vi "GET Save Directory.vi"() -> (0 "Save Directory":path)   [LabVIEW 2013]
uses:
  Action.ctl
  Persistent Data FGV Selector.ctl
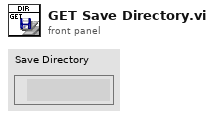
[diagram p1: front panel]
types:
  T1 = typedef "Persistent Data FGV Selector.ctl" = enum16{"Save Directory", "File Name"}
  T2 = typedef "Action.ctl" = enum16{"GET", "PUT", "DELETE"}
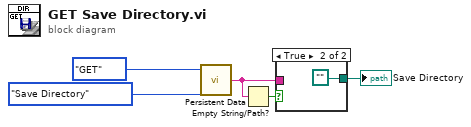
[diagram p0: block diagram]
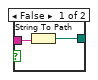
[diagram p2: hidden frame]
diagram:
  n1 = call "Persistent Data.vi"("Persistent Data FGV Selector"=Persistent_Data_FGV_Selector."Save Directory", "Action"=Action."GET") -> ("Output"=w1:string)  [unwired: 1 in]
  n2 = Empty String/Path?(string/path=w1) -> (empty?=w2:bool)
  n3 = case shown="True" w2 {
    tunnel: w1 -> [w7 _]
    tunnel: [w6 path ""] -> w3
    frame False {
      n4 = String To Path(string=w7) -> (path=w6:path)
    }
    frame True {
    }
  }
  "Save Directory" <- w3
